vi "Autonomous Independent.vi"() -> ()   [LabVIEW 2018]
doc: "This VI is called when autonomous begins, and will automatically be terminated when autonomous ends. You can carry out timed or sensor driven robot movement independently without needing to return to the caller."
uses:
  <vilib>/Rock Robotics/WPI/Utilities/WPI_GetSetVariantRefNum.vi
  <vilib>/Rock Robotics/Network Tables/NT Read String.vi
  <vilib>/Rock Robotics/Network Tables/NT Write Numeric Array.vi
  <vilib>/Rock Robotics/WPI/RobotDrive/WPI_RobotDriveArcadeDrive_Standard(NoSaturation).vi
panel:
  out "Current Movement, for debugging":T1 {"Y Joystick Value" scale=1.0..-1.0; "X Joystick Value" scale=-1.0..1.0}
  in  "Array of robot movements":T2(array[cluster])=[{"X Joystick Value"=0.39393939393939403, "Y Joystick Value"=0.0, "Delay (sec)"=1.0, "Movement Name"="turn"}, {"X Joystick Value"=-0.3737373737373737, "Y Joystick Value"=0.0, "Delay (sec)"=1.0, "Movement Name"="turn back"}] {"Y Joystick Value" scale=1.0..-1.0; "X Joystick Value" scale=-1.0..1.0}
  # "Be sure to right-click and choose Data Operations>>Make Current Value default if you want to save the array values with the VI"
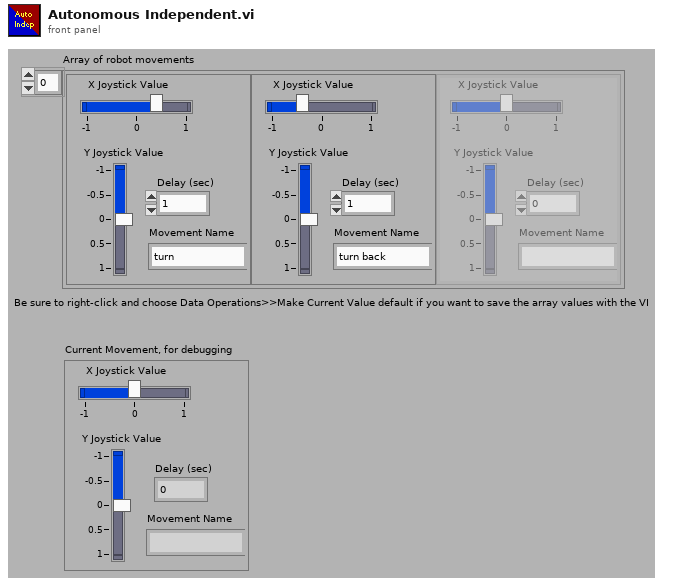
[diagram p1: front panel]
types:
  T1 = cluster{"X Joystick Value":dbl, "Y Joystick Value":dbl, "Delay (sec)":dbl, "Movement Name":string}
  T2 = cluster{"X Joystick Value":dbl, "Y Joystick Value":dbl, "Delay (sec)":dbl, "Movement Name":string}[]
  T3 = typedef "WPI_JoystickDevRef.ctl" = cluster{"Device":T4}
  T4 = typedef "WPI_JoystickDeviceEnum.ctl" = enum16{"USB 0", "USB 1", "USB 2", "USB 3", "USB 4", "USB 5"}
  T5 = typedef "WPI_RobotDriveDevRef.ctl" = cluster{"DevStatus":errorcluster, "Motors[]":T6[], "Square Inputs":bool, "Max Output":dbl}
  T6 = typedef "WPI_MotorControlDeviceRef.ctl" = cluster{"DeviceStatus":errorcluster, "Type":T7, "PWM":cluster{"PWM Channel":T8, "DeadBand":T9}, "CAN":cluster{"Device Number":u8, "SetOutput VI Ref":variant, "GetOutput VI Ref":variant, "Enable VI Ref":variant, "Disable VI Ref":variant, "Data":variant}, "Invert":bool, "DIO PWM":cluster{"PWM \"Enable\" Channel":T8, "DIOChannel":T10, "PWM Rate":dbl}}
  T7 = typedef "WPI_MotorControlType.ctl" = enum16{"PWM", "CAN", "DIO PWM"}
  T8 = typedef "FPGA_DIOPWMChannel.ctl" = enum8{"PWM 0", "PWM 1", "PWM 2", "PWM 3", "PWM 4", "PWM 5", "PWM 6", "PWM 7", "PWM 8", "PWM 9", "PWM MXP 0", "PWM MXP 1", "PWM MXP 2", "PWM MXP 3", "PWM MXP 4", "PWM MXP 5", "PWM MXP 6", "PWM MXP 7", "PWM MXP 8", "PWM MXP 9", "Invalid"}
  T9 = typedef "WPI_PWMDeadband.ctl" = cluster{"Name":string, "maxPositivePwm":i32, "minPositivePwm":i32, "centerPwm":i32, "maxNegativePwm":i32, "minNegativePwm":i32, "angularRange":u16}
  T10 = typedef "FPGA_DIOChannel.ctl" = enum8{"DIO 0", "DIO 1", "DIO 2", "DIO 3", "DIO 4", "DIO 5", "DIO 6", "DIO 7", "DIO 8", "DIO 9", "DIO MXP 0", "DIO MXP 1", "DIO MXP 2", "DIO MXP 3", "DIO MXP 4", "DIO MXP 5", "DIO MXP 6", "DIO MXP 7", "DIO MXP 8", "DIO MXP 9", "DIO MXP 10", "DIO MXP 11", "DIO MXP 12", "DIO MXP 13", "DIO MXP 14", "DIO MXP 15", "SPI Port CS1", "SPI Port CS2", "SPI Port CS3", "SPI Port MISO", "SPI Port MOSI", "Invalid"}
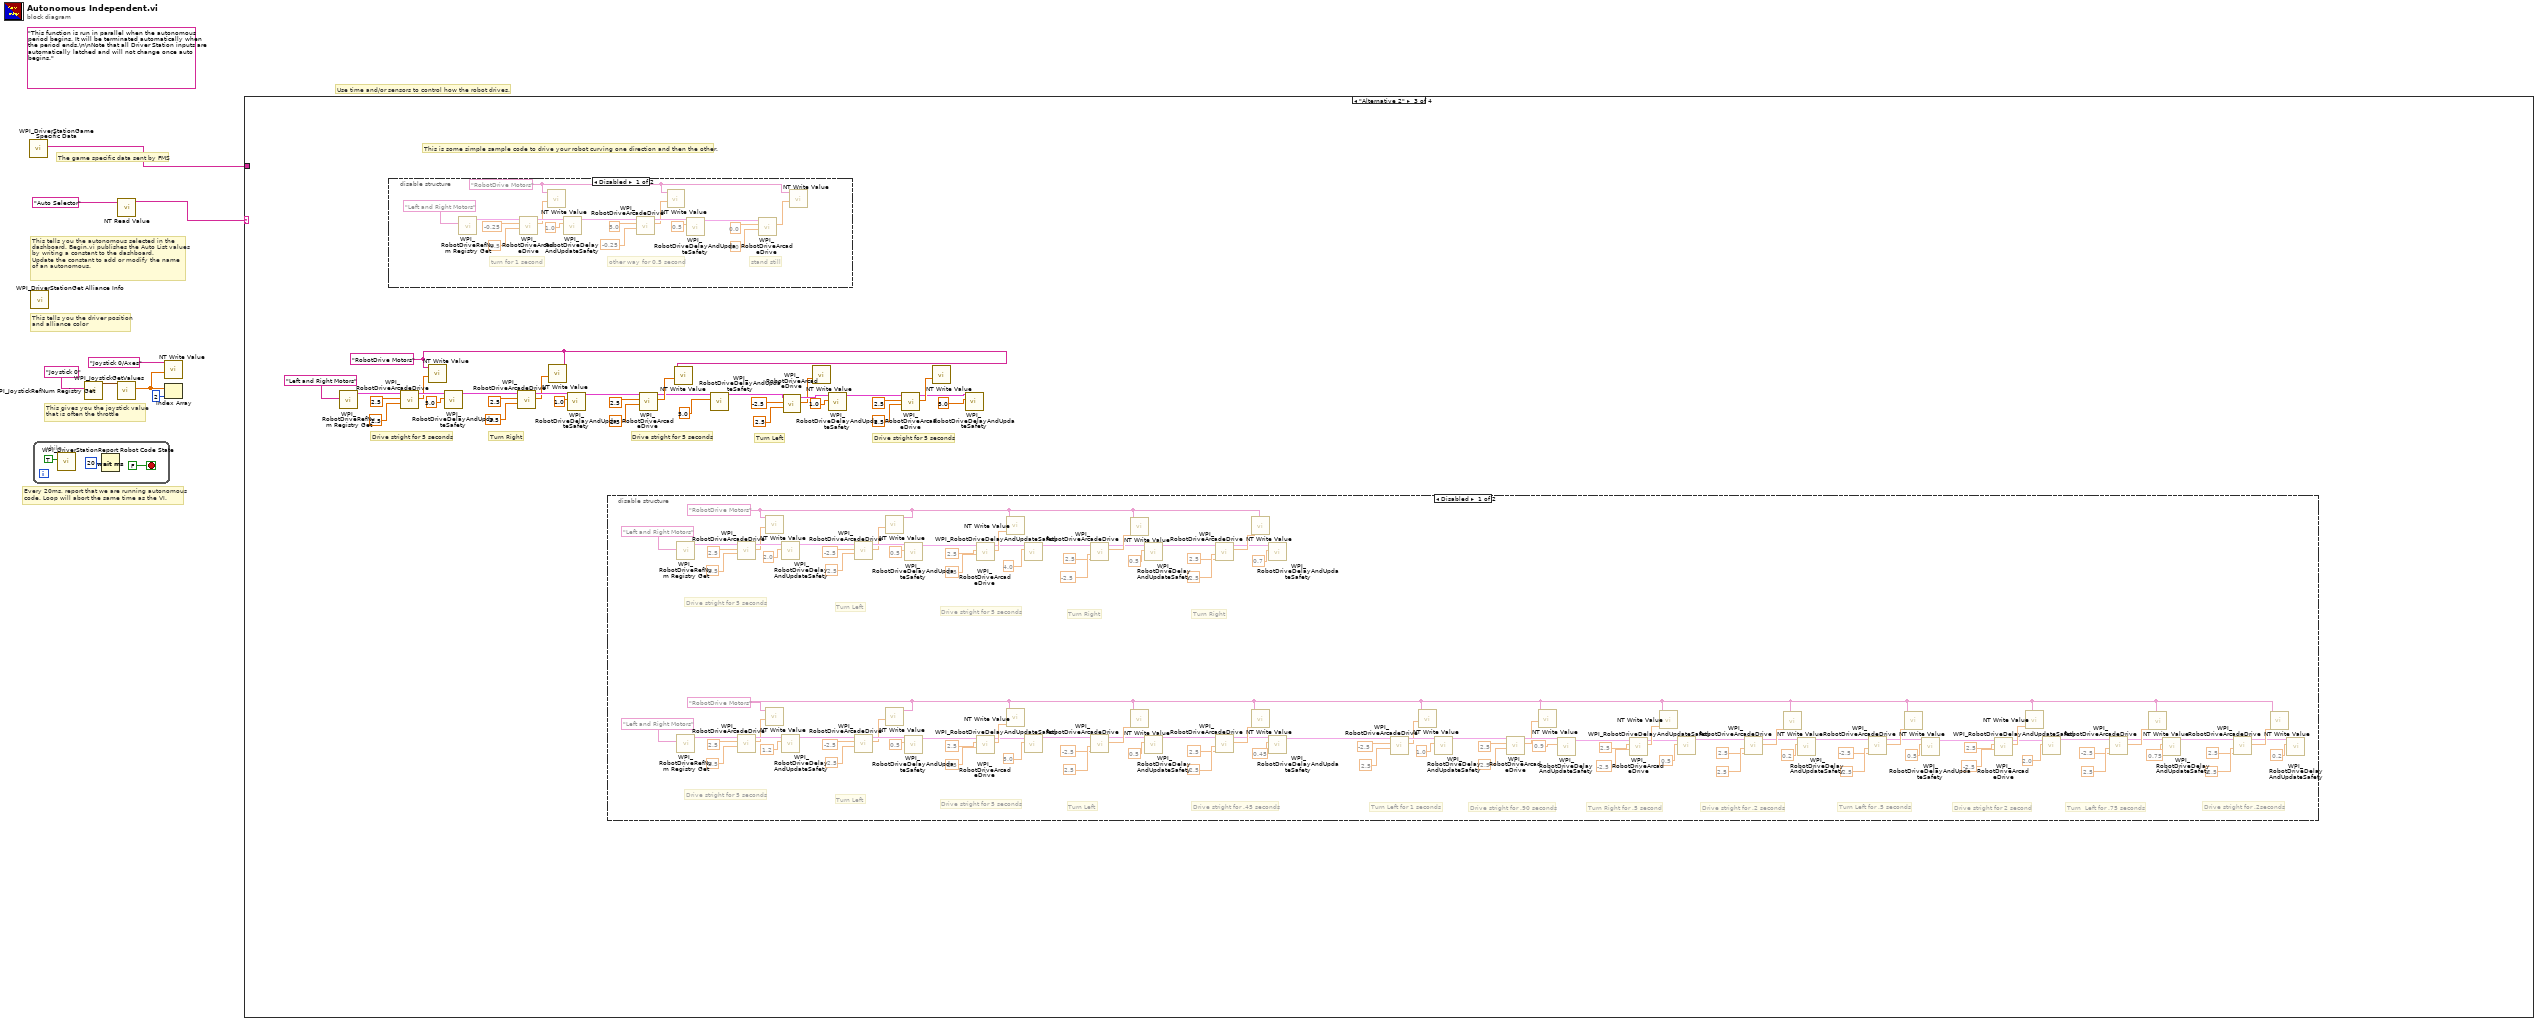
[diagram p0: block diagram]
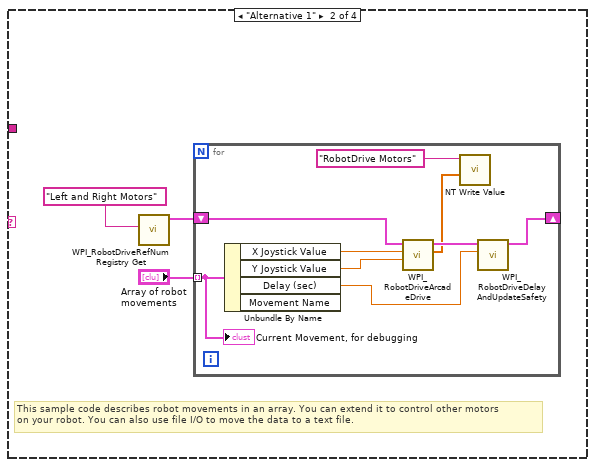
[diagram p3: hidden frame]
diagram:
  (unwired) "This function is run in parallel when the autonomous period begins. It will be terminated automatically when the period ends.\n\nNote that all Driver Station inputs are automatically latched and will not change once auto begins."
  # "The game specific data sent by FMS"
  # "This tells you the autonomous selected in the \ndashboard. Begin.vi publishes the Auto List values\nby writing a constant to the dashboard.\nUpdate the constant to add or modify the name\nof an autonomous."
  # "Every 20ms, report that we are running autonomous\ncode. Loop will abort the same time as the VI."
  # "This gives you the joystick value\nthat is often the throttle"
  # "Use time and/or sensors to control how the robot drives."
  # "This tells you the driver position\nand alliance color"
  n1 = call <vilib>:"WPI_DriverStationGame Specific Data.vi"() -> ("Game Specific Data"=w1:string)  [unwired: 11 in]
  n2 = call <vilib>:"WPI_DriverStationGet Alliance Info.vi"() -> ()  [unwired: 12 out]
  n3 = while {
    stop <- FALSE stop-if-true
    n4 = call <vilib>:"WPI_DriverStationReport Robot Code State.vi"("Autonomous"=TRUE) -> ()  [unwired: 10 in, 1 out]
    n5 = Wait (ms)(milliseconds to wait=u32 20) -> ()  [unwired: 1 out]
  }
  n6 = call <vilib>:"WPI_JoystickRefNum Registry Get.vi"("refnum name"="Joystick 0") -> ("JoystickDevRef"=w7:T3)  [unwired: 1 in, 9 out]
  n7 = call <vilib>:"WPI_JoystickGetValues.vi"("JoystickDevRef"=w7) -> ("Axes"=w3:dbl[])  [unwired: 6 in, 4 out]
  n8 = call-poly <vilib>:"NT Read Value.vi"("Name"="Auto Selector") -> ("String"=w4:string)  [unwired: 9 in, 1 out]
  n9 = call-poly <vilib>:"NT Write Value.vi"("Numeric Array"=w3, "Name"="Joystick 0/Axes") -> ()  [unwired: 9 in, 1 out]
  n10 = Index Array(array=w3, index=2) -> ()  [unwired: 1 out]
  n11 = case shown="\"Alternative 2\"" w4 {
    tunnel: w1 -> [_ _ _ _]
    frame Default {
      # "You can put your main auto here, or you can right-click on the case and make any\nother frame be the default case."
      # "This is the frame that will execute if no selection is made, or if it is not recognized"
    }
    frame "Alternative 1" {
      # "This sample code describes robot movements in an array. You can extend it to control other motors\non your robot. You can also use file I/O to move the data to a text file."
      n12 = call <vilib>:"WPI_RobotDriveRefNum Registry Get.vi"("refnum name"="Left and Right Motors") -> ("RobotDriveDevRef"=w13:T5)  [unwired: 1 in, 9 out]
      n13 = for {
        shift-right: [w21] -> _
        shift-left: w13 -> [w22]
        tunnel: "Array of robot movements" -> [w17] mode=indexing
        n14 = Unbundle By Name(w17) -> ("X Joystick Value"=w20:dbl, "Y Joystick Value"=w19:dbl, "Delay (sec)"=w18:dbl)  [unwired: 1 out]
        n15 = call-poly <vilib>:"WPI_RobotDriveArcadeDrive.vi"("Y axis value"=w19, "X axis value"=w20, "RobotDriveDevRef"=w22) -> ("Motor Values"=w15:dbl[], "RobotDriveDevRef"=w23:T5)  [unwired: 1 in, 6 out]
        n16 = call-poly <vilib>:"NT Write Value.vi"("Numeric Array"=w15, "Name"="RobotDrive Motors") -> ()  [unwired: 9 in, 1 out]
        n17 = call <vilib>:"WPI_RobotDriveDelayAndUpdateSafety.vi"("Delay (s)"=w18, "RobotDriveDevRef"=w23) -> ("RobotDriveDevRef 2"=w21:T5)  [unwired: 8 in, 1 out]
        "Current Movement, for debugging" <- w17
      }
    }
    frame "Alternative 2" {
      w39 = "RobotDrive Motors" ("Name")
      # "Drive stright for 5 seconds"
      # "Turn Left"
      # "Drive stright for 5 seconds"
      # "Turn Right"
      # "Drive stright for 5 seconds"
      # "This is some simple sample code to drive your robot curving one direction and then the other."
      n18 = call <vilib>:"WPI_RobotDriveRefNum Registry Get.vi"("refnum name"="Left and Right Motors") -> ("RobotDriveDevRef"=w55:T5)  [unwired: 1 in, 9 out]
      n19 = disable-structure shown="Disabled" {
        frame Disabled {
          w169 = "RobotDrive Motors" ("Name")
          # "stand still"
          # "other way for 0.5 second"
          # "turn for 1 second"
          n20 = call <vilib>:"WPI_RobotDriveRefNum Registry Get.vi"("refnum name"="Left and Right Motors") -> ("RobotDriveDevRef"=w185:T5)  [unwired: 1 in, 9 out]
          n21 = call-poly <vilib>:"WPI_RobotDriveArcadeDrive.vi"("Y axis value"=0.5 ("X axis value"), "X axis value"=-0.25, "RobotDriveDevRef"=w185) -> ("Motor Values"=w168:dbl[], "RobotDriveDevRef"=w178:T5)  [unwired: 1 in, 6 out]
          n22 = call-poly <vilib>:"NT Write Value.vi"("Numeric Array"=w168, "Name"=w169) -> ()  [unwired: 9 in, 1 out]
          n23 = call <vilib>:"WPI_RobotDriveDelayAndUpdateSafety.vi"("Delay (s)"=1.0, "RobotDriveDevRef"=w178) -> ("RobotDriveDevRef 2"=w179:T5)  [unwired: 8 in, 1 out]
          n24 = call-poly <vilib>:"WPI_RobotDriveArcadeDrive.vi"("Y axis value"=-0.25 ("X axis value"), "X axis value"=5.0, "RobotDriveDevRef"=w179) -> ("Motor Values"=w170:dbl[], "RobotDriveDevRef"=w180:T5)  [unwired: 1 in, 6 out]
          n25 = call-poly <vilib>:"NT Write Value.vi"("Numeric Array"=w170, "Name"=w169) -> ()  [unwired: 9 in, 1 out]
          n26 = call <vilib>:"WPI_RobotDriveDelayAndUpdateSafety.vi"("Delay (s)"=0.5, "RobotDriveDevRef"=w180) -> ("RobotDriveDevRef 2"=w181:T5)  [unwired: 8 in, 1 out]
          n27 = call-poly <vilib>:"WPI_RobotDriveArcadeDrive.vi"("Y axis value"=0.0 ("X axis value"), "X axis value"=0.0, "RobotDriveDevRef"=w181) -> ("Motor Values"=w171:dbl[])  [unwired: 1 in, 7 out]
          n28 = call-poly <vilib>:"NT Write Value.vi"("Numeric Array"=w171, "Name"=w169) -> ()  [unwired: 9 in, 1 out]
        }
        frame Enabled {
        }
      }
      n29 = call-poly <vilib>:"WPI_RobotDriveArcadeDrive.vi"("Y axis value"=2.5 ("X axis value"), "X axis value"=2.5, "RobotDriveDevRef"=w55) -> ("Motor Values"=w38:dbl[], "RobotDriveDevRef"=w48:T5)  [unwired: 1 in, 6 out]
      n30 = call-poly <vilib>:"NT Write Value.vi"("Numeric Array"=w38, "Name"=w39) -> ()  [unwired: 9 in, 1 out]
      n31 = call <vilib>:"WPI_RobotDriveDelayAndUpdateSafety.vi"("Delay (s)"=5.0, "RobotDriveDevRef"=w48) -> ("RobotDriveDevRef 2"=w49:T5)  [unwired: 8 in, 1 out]
      n32 = call-poly <vilib>:"WPI_RobotDriveArcadeDrive.vi"("Y axis value"=-2.5 ("X axis value"), "X axis value"=2.5, "RobotDriveDevRef"=w49) -> ("Motor Values"=w40:dbl[], "RobotDriveDevRef"=w50:T5)  [unwired: 1 in, 6 out]
      n33 = call-poly <vilib>:"NT Write Value.vi"("Numeric Array"=w40, "Name"=w39) -> ()  [unwired: 9 in, 1 out]
      n34 = call <vilib>:"WPI_RobotDriveDelayAndUpdateSafety.vi"("Delay (s)"=1.0, "RobotDriveDevRef"=w50) -> ("RobotDriveDevRef 2"=w51:T5)  [unwired: 8 in, 1 out]
      n35 = disable-structure shown="Disabled" {
        frame Disabled {
          w57 = "RobotDrive Motors" ("Name")
          w136 = "RobotDrive Motors" ("Name")
          # "Drive stright for .2seconds"
          # "Turn  Left for .75 seconds"
          # "Drive stright for 2 second"
          # "Turn Left for .5 seconds"
          # "Drive stright for .2 seconds"
          # "Turn Right for .5 second"
          # "Drive stright for .90 seconds"
          # "Turn Left for 1 seconds"
          # "Drive stright for .45 seconds"
          # "Drive stright for 5 seconds"
          # "Turn Left"
          # "Turn Left"
          # "Drive stright for 5 seconds"
          # "Turn Right"
          # "Drive stright for 5 seconds"
          # "Turn Right"
          # "Turn Left"
          # "Drive stright for 5 seconds"
          n36 = call <vilib>:"WPI_RobotDriveRefNum Registry Get.vi"("refnum name"="Left and Right Motors") -> ("RobotDriveDevRef"=w167:T5)  [unwired: 1 in, 9 out]
          n37 = call <vilib>:"WPI_RobotDriveRefNum Registry Get.vi"("refnum name"="Left and Right Motors") -> ("RobotDriveDevRef"=w135:T5)  [unwired: 1 in, 9 out]
          n38 = call-poly <vilib>:"WPI_RobotDriveArcadeDrive.vi"("Y axis value"=2.5 ("X axis value"), "X axis value"=2.5, "RobotDriveDevRef"=w167) -> ("Motor Values"=w152:dbl[], "RobotDriveDevRef"=w160:T5)  [unwired: 1 in, 6 out]
          n39 = call-poly <vilib>:"WPI_RobotDriveArcadeDrive.vi"("Y axis value"=2.5 ("X axis value"), "X axis value"=2.5, "RobotDriveDevRef"=w135) -> ("Motor Values"=w120:dbl[], "RobotDriveDevRef"=w128:T5)  [unwired: 1 in, 6 out]
          n40 = call-poly <vilib>:"NT Write Value.vi"("Numeric Array"=w152, "Name"=w136) -> ()  [unwired: 9 in, 1 out]
          n41 = call-poly <vilib>:"NT Write Value.vi"("Numeric Array"=w120, "Name"=w57) -> ()  [unwired: 9 in, 1 out]
          n42 = call <vilib>:"WPI_RobotDriveDelayAndUpdateSafety.vi"("Delay (s)"=2.0, "RobotDriveDevRef"=w160) -> ("RobotDriveDevRef 2"=w161:T5)  [unwired: 8 in, 1 out]
          n43 = call <vilib>:"WPI_RobotDriveDelayAndUpdateSafety.vi"("Delay (s)"=1.2, "RobotDriveDevRef"=w128) -> ("RobotDriveDevRef 2"=w129:T5)  [unwired: 8 in, 1 out]
          n44 = call-poly <vilib>:"WPI_RobotDriveArcadeDrive.vi"("Y axis value"=2.5 ("X axis value"), "X axis value"=-2.5, "RobotDriveDevRef"=w161) -> ("Motor Values"=w153:dbl[], "RobotDriveDevRef"=w162:T5)  [unwired: 1 in, 6 out]
          n45 = call-poly <vilib>:"WPI_RobotDriveArcadeDrive.vi"("Y axis value"=2.5 ("X axis value"), "X axis value"=-2.5, "RobotDriveDevRef"=w129) -> ("Motor Values"=w121:dbl[], "RobotDriveDevRef"=w130:T5)  [unwired: 1 in, 6 out]
          n46 = call-poly <vilib>:"NT Write Value.vi"("Numeric Array"=w153, "Name"=w136) -> ()  [unwired: 9 in, 1 out]
          n47 = call-poly <vilib>:"NT Write Value.vi"("Numeric Array"=w121, "Name"=w57) -> ()  [unwired: 9 in, 1 out]
          n48 = call <vilib>:"WPI_RobotDriveDelayAndUpdateSafety.vi"("Delay (s)"=0.5, "RobotDriveDevRef"=w162) -> ("RobotDriveDevRef 2"=w163:T5)  [unwired: 8 in, 1 out]
          n49 = call <vilib>:"WPI_RobotDriveDelayAndUpdateSafety.vi"("Delay (s)"=0.5, "RobotDriveDevRef"=w130) -> ("RobotDriveDevRef 2"=w131:T5)  [unwired: 8 in, 1 out]
          n50 = call-poly <vilib>:"WPI_RobotDriveArcadeDrive.vi"("Y axis value"=2.5 ("X axis value"), "X axis value"=2.5, "RobotDriveDevRef"=w163) -> ("Motor Values"=w154:dbl[], "RobotDriveDevRef"=w150:T5)  [unwired: 1 in, 6 out]
          n51 = call-poly <vilib>:"WPI_RobotDriveArcadeDrive.vi"("Y axis value"=2.5 ("X axis value"), "X axis value"=2.5, "RobotDriveDevRef"=w131) -> ("Motor Values"=w122:dbl[], "RobotDriveDevRef"=w118:T5)  [unwired: 1 in, 6 out]
          n52 = call-poly <vilib>:"NT Write Value.vi"("Numeric Array"=w154, "Name"=w136) -> ()  [unwired: 9 in, 1 out]
          n53 = call-poly <vilib>:"NT Write Value.vi"("Numeric Array"=w122, "Name"=w57) -> ()  [unwired: 9 in, 1 out]
          n54 = call <vilib>:"WPI_RobotDriveDelayAndUpdateSafety.vi"("Delay (s)"=4.0, "RobotDriveDevRef"=w150) -> ("RobotDriveDevRef 2"=w144:T5)  [unwired: 8 in, 1 out]
          n55 = call <vilib>:"WPI_RobotDriveDelayAndUpdateSafety.vi"("Delay (s)"=5.0, "RobotDriveDevRef"=w118) -> ("RobotDriveDevRef 2"=w112:T5)  [unwired: 8 in, 1 out]
          n56 = call-poly <vilib>:"WPI_RobotDriveArcadeDrive.vi"("Y axis value"=-2.5 ("X axis value"), "X axis value"=2.5, "RobotDriveDevRef"=w144) -> ("Motor Values"=w148:dbl[], "RobotDriveDevRef"=w146:T5)  [unwired: 1 in, 6 out]
          n57 = call-poly <vilib>:"WPI_RobotDriveArcadeDrive.vi"("Y axis value"=2.5 ("X axis value"), "X axis value"=-2.5, "RobotDriveDevRef"=w112) -> ("Motor Values"=w116:dbl[], "RobotDriveDevRef"=w114:T5)  [unwired: 1 in, 6 out]
          n58 = call-poly <vilib>:"NT Write Value.vi"("Numeric Array"=w148, "Name"=w136) -> ()  [unwired: 9 in, 1 out]
          n59 = call-poly <vilib>:"NT Write Value.vi"("Numeric Array"=w116, "Name"=w57) -> ()  [unwired: 9 in, 1 out]
          n60 = call <vilib>:"WPI_RobotDriveDelayAndUpdateSafety.vi"("Delay (s)"=0.5, "RobotDriveDevRef"=w146) -> ("RobotDriveDevRef 2"=w137:T5)  [unwired: 8 in, 1 out]
          n61 = call <vilib>:"WPI_RobotDriveDelayAndUpdateSafety.vi"("Delay (s)"=0.5, "RobotDriveDevRef"=w114) -> ("RobotDriveDevRef 2"=w105:T5)  [unwired: 8 in, 1 out]
          n62 = call-poly <vilib>:"WPI_RobotDriveArcadeDrive.vi"("Y axis value"=2.5 ("X axis value"), "X axis value"=2.5, "RobotDriveDevRef"=w137) -> ("Motor Values"=w141:dbl[], "RobotDriveDevRef"=w139:T5)  [unwired: 1 in, 6 out]
          n63 = call-poly <vilib>:"WPI_RobotDriveArcadeDrive.vi"("Y axis value"=2.5 ("X axis value"), "X axis value"=2.5, "RobotDriveDevRef"=w105) -> ("Motor Values"=w109:dbl[], "RobotDriveDevRef"=w107:T5)  [unwired: 1 in, 6 out]
          n64 = call-poly <vilib>:"NT Write Value.vi"("Numeric Array"=w141, "Name"=w136) -> ()  [unwired: 9 in, 1 out]
          n65 = call-poly <vilib>:"NT Write Value.vi"("Numeric Array"=w109, "Name"=w57) -> ()  [unwired: 9 in, 1 out]
          n66 = call <vilib>:"WPI_RobotDriveDelayAndUpdateSafety.vi"("Delay (s)"=0.7, "RobotDriveDevRef"=w139) -> ()  [unwired: 8 in, 2 out]
          n67 = call <vilib>:"WPI_RobotDriveDelayAndUpdateSafety.vi"("Delay (s)"=0.45, "RobotDriveDevRef"=w107) -> ("RobotDriveDevRef 2"=w75:T5)  [unwired: 8 in, 1 out]
          n68 = call-poly <vilib>:"WPI_RobotDriveArcadeDrive.vi"("Y axis value"=2.5 ("X axis value"), "X axis value"=-2.5, "RobotDriveDevRef"=w75) -> ("Motor Values"=w91:dbl[], "RobotDriveDevRef"=w99:T5)  [unwired: 1 in, 6 out]
          n69 = call-poly <vilib>:"NT Write Value.vi"("Numeric Array"=w91, "Name"=w57) -> ()  [unwired: 9 in, 1 out]
          n70 = call <vilib>:"WPI_RobotDriveDelayAndUpdateSafety.vi"("Delay (s)"=1.0, "RobotDriveDevRef"=w99) -> ("RobotDriveDevRef 2"=w100:T5)  [unwired: 8 in, 1 out]
          n71 = call-poly <vilib>:"WPI_RobotDriveArcadeDrive.vi"("Y axis value"=2.5 ("X axis value"), "X axis value"=2.5, "RobotDriveDevRef"=w100) -> ("Motor Values"=w92:dbl[], "RobotDriveDevRef"=w101:T5)  [unwired: 1 in, 6 out]
          n72 = call-poly <vilib>:"NT Write Value.vi"("Numeric Array"=w92, "Name"=w57) -> ()  [unwired: 9 in, 1 out]
          n73 = call <vilib>:"WPI_RobotDriveDelayAndUpdateSafety.vi"("Delay (s)"=0.9, "RobotDriveDevRef"=w101) -> ("RobotDriveDevRef 2"=w102:T5)  [unwired: 8 in, 1 out]
          n74 = call-poly <vilib>:"WPI_RobotDriveArcadeDrive.vi"("Y axis value"=-2.5 ("X axis value"), "X axis value"=2.5, "RobotDriveDevRef"=w102) -> ("Motor Values"=w93:dbl[], "RobotDriveDevRef"=w89:T5)  [unwired: 1 in, 6 out]
          n75 = call-poly <vilib>:"NT Write Value.vi"("Numeric Array"=w93, "Name"=w57) -> ()  [unwired: 9 in, 1 out]
          n76 = call <vilib>:"WPI_RobotDriveDelayAndUpdateSafety.vi"("Delay (s)"=0.5, "RobotDriveDevRef"=w89) -> ("RobotDriveDevRef 2"=w83:T5)  [unwired: 8 in, 1 out]
          n77 = call-poly <vilib>:"WPI_RobotDriveArcadeDrive.vi"("Y axis value"=2.5 ("X axis value"), "X axis value"=2.5, "RobotDriveDevRef"=w83) -> ("Motor Values"=w87:dbl[], "RobotDriveDevRef"=w85:T5)  [unwired: 1 in, 6 out]
          n78 = call-poly <vilib>:"NT Write Value.vi"("Numeric Array"=w87, "Name"=w57) -> ()  [unwired: 9 in, 1 out]
          n79 = call <vilib>:"WPI_RobotDriveDelayAndUpdateSafety.vi"("Delay (s)"=0.2, "RobotDriveDevRef"=w85) -> ("RobotDriveDevRef 2"=w76:T5)  [unwired: 8 in, 1 out]
          n80 = call-poly <vilib>:"WPI_RobotDriveArcadeDrive.vi"("Y axis value"=2.5 ("X axis value"), "X axis value"=-2.5, "RobotDriveDevRef"=w76) -> ("Motor Values"=w80:dbl[], "RobotDriveDevRef"=w78:T5)  [unwired: 1 in, 6 out]
          n81 = call-poly <vilib>:"NT Write Value.vi"("Numeric Array"=w80, "Name"=w57) -> ()  [unwired: 9 in, 1 out]
          n82 = call <vilib>:"WPI_RobotDriveDelayAndUpdateSafety.vi"("Delay (s)"=0.5, "RobotDriveDevRef"=w78) -> ("RobotDriveDevRef 2"=w56:T5)  [unwired: 8 in, 1 out]
          n83 = call-poly <vilib>:"WPI_RobotDriveArcadeDrive.vi"("Y axis value"=-2.5 ("X axis value"), "X axis value"=2.5, "RobotDriveDevRef"=w56) -> ("Motor Values"=w73:dbl[], "RobotDriveDevRef"=w71:T5)  [unwired: 1 in, 6 out]
          n84 = call-poly <vilib>:"NT Write Value.vi"("Numeric Array"=w73, "Name"=w57) -> ()  [unwired: 9 in, 1 out]
          n85 = call <vilib>:"WPI_RobotDriveDelayAndUpdateSafety.vi"("Delay (s)"=2.0, "RobotDriveDevRef"=w71) -> ("RobotDriveDevRef 2"=w65:T5)  [unwired: 8 in, 1 out]
          n86 = call-poly <vilib>:"WPI_RobotDriveArcadeDrive.vi"("Y axis value"=2.5 ("X axis value"), "X axis value"=-2.5, "RobotDriveDevRef"=w65) -> ("Motor Values"=w69:dbl[], "RobotDriveDevRef"=w67:T5)  [unwired: 1 in, 6 out]
          n87 = call-poly <vilib>:"NT Write Value.vi"("Numeric Array"=w69, "Name"=w57) -> ()  [unwired: 9 in, 1 out]
          n88 = call <vilib>:"WPI_RobotDriveDelayAndUpdateSafety.vi"("Delay (s)"=0.75, "RobotDriveDevRef"=w67) -> ("RobotDriveDevRef 2"=w58:T5)  [unwired: 8 in, 1 out]
          n89 = call-poly <vilib>:"WPI_RobotDriveArcadeDrive.vi"("Y axis value"=2.5 ("X axis value"), "X axis value"=2.5, "RobotDriveDevRef"=w58) -> ("Motor Values"=w62:dbl[], "RobotDriveDevRef"=w60:T5)  [unwired: 1 in, 6 out]
          n90 = call-poly <vilib>:"NT Write Value.vi"("Numeric Array"=w62, "Name"=w57) -> ()  [unwired: 9 in, 1 out]
          n91 = call <vilib>:"WPI_RobotDriveDelayAndUpdateSafety.vi"("Delay (s)"=0.2, "RobotDriveDevRef"=w60) -> ()  [unwired: 8 in, 2 out]
        }
        frame Enabled {
        }
      }
      n92 = call-poly <vilib>:"WPI_RobotDriveArcadeDrive.vi"("Y axis value"=2.5 ("X axis value"), "X axis value"=2.5, "RobotDriveDevRef"=w51) -> ("Motor Values"=w41:dbl[], "RobotDriveDevRef"=w27:T5)  [unwired: 1 in, 6 out]
      n93 = call-poly <vilib>:"NT Write Value.vi"("Numeric Array"=w41, "Name"=w39) -> ()  [unwired: 9 in, 1 out]
      n94 = call <vilib>:"WPI_RobotDriveDelayAndUpdateSafety.vi"("Delay (s)"=5.0, "RobotDriveDevRef"=w27) -> ("RobotDriveDevRef 2"=w26:T5)  [unwired: 8 in, 1 out]
      n95 = call-poly <vilib>:"WPI_RobotDriveArcadeDrive.vi"("Y axis value"=2.5 ("X axis value"), "X axis value"=-2.5, "RobotDriveDevRef"=w26) -> ("Motor Values"=w29:dbl[], "RobotDriveDevRef"=w35:T5)  [unwired: 1 in, 6 out]
      n96 = call-poly <vilib>:"NT Write Value.vi"("Numeric Array"=w29) -> ()  [unwired: 10 in, 1 out]
      n97 = call <vilib>:"WPI_RobotDriveDelayAndUpdateSafety.vi"("Delay (s)"=1.0, "RobotDriveDevRef"=w35) -> ("RobotDriveDevRef 2"=w36:T5)  [unwired: 8 in, 1 out]
      n98 = call-poly <vilib>:"WPI_RobotDriveArcadeDrive.vi"("Y axis value"=2.5 ("X axis value"), "X axis value"=2.5, "RobotDriveDevRef"=w36) -> ("Motor Values"=w30:dbl[], "RobotDriveDevRef"=w24:T5)  [unwired: 1 in, 6 out]
      n99 = call-poly <vilib>:"NT Write Value.vi"("Numeric Array"=w30) -> ()  [unwired: 10 in, 1 out]
      n100 = call <vilib>:"WPI_RobotDriveDelayAndUpdateSafety.vi"("Delay (s)"=5.0, "RobotDriveDevRef"=w24) -> ()  [unwired: 8 in, 2 out]
    }
    frame "Your Turn" {
    }
  }
